vi "Draw Frame.vi"(8 "Error In":errorcluster, 11 "Display In":refnum<class "Display.lvclass">) -> (0 "Error Out":errorcluster, 2 "Frame":u32[][](array[colorbox]), 3 "Display Out":refnum<class "Display.lvclass">)   [LabVIEW 2019, in "Display.lvclass"]
uses:
  Display.lvclass
  Display Element/Display Element.lvclass
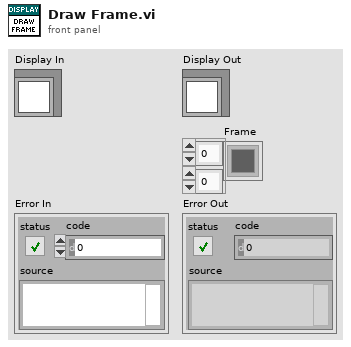
[diagram p1: front panel]
types:
  T1 = typedef "Display Element.lvclass/Pixel.ctl" = cluster{"Position":T2, "Color":u32}
  T2 = typedef "Display Element.lvclass/Vector.ctl" = cluster{"X":i32, "Y":i32}
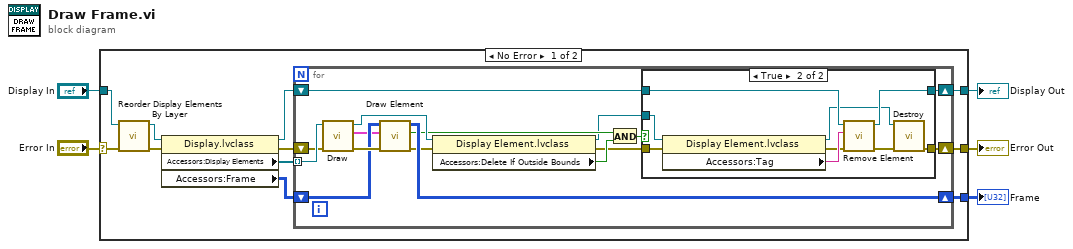
[diagram p0: block diagram]
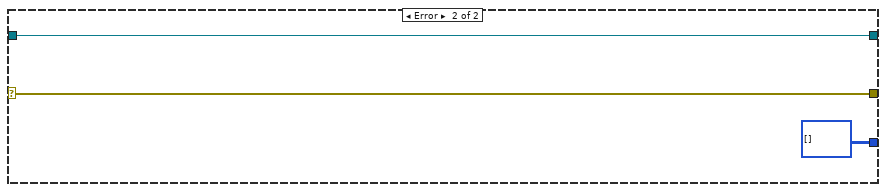
[diagram p3: hidden frame]
diagram:
  n1 = case shown="No Error" "Error In" {
    selector: "Error In" -> [w7 w45]
    tunnel: "Display In" -> [w6 w46]
    tunnel: [w11 w46] -> w3
    tunnel: [w13 w45] -> w2
    tunnel: [w14 u32[][] [] ("Accessors:Frame")] -> w1
    frame No Error {
      n2 = call "Reorder Display Elements By Layer.vi"("Error In"=w7, "Display In"=w6) -> ("Error Out"=w8:errorcluster, "Display Out"=w9:refnum<class "Display.lvclass">)  [unwired: 8 in]
      n3 = property class="Display.lvclass"(reference=w9, error in=w8) -> (reference out=w12:refnum<class "Display.lvclass">, error out=w15:errorcluster, "Accessors:Display Elements"=w16:refnum<class "Display Element.lvclass">[], "Accessors:Frame"=w10:u32[][])
      n4 = for {
        tunnel: w16 -> [w32] mode=indexing
        shift-right: [w28] -> w13
        shift-left: w15 -> [w31]
        shift-right: [w29] -> w14
        shift-left: w10 -> [w25]
        shift-right: [w26] -> w11
        shift-left: w12 -> [w27]
        n5 = call-dynamic "Draw.vi"("Error In"=w31, "Display Element In"=w32) -> ("Error Out"=w30:errorcluster, "Element To Display"=w24:T1[], "Display Element Out"=w23:refnum<class "Display Element.lvclass">)  [unwired: 7 in]
        n6 = call "Draw Element.vi"("Error In"=w30, "Element To Display"=w24, "Frame In"=w25) -> ("Error Out"=w22:errorcluster, "Frame Changed?"=w21:bool, "Frame Out"=w29:u32[][])  [unwired: 6 in]
        n7 = property class="Display Element.lvclass"(reference=w23, error in=w22) -> (reference out=w19:refnum<class "Display Element.lvclass">, error out=w17:errorcluster, "Accessors:Delete If Outside Bounds"=w20:bool)
        n8 = And(x=w21, y=w20) -> (x .and. y?=w18:bool)
        n9 = case shown="True" w18 {
          tunnel: [w33 w42] -> w28
          tunnel: w27 -> [w34 w41]
          tunnel: [w34 w40] -> w26
          tunnel: w19 -> [_ w39]
          tunnel: w17 -> [w33 w38]
          frame False {
          }
          frame True {
            n10 = property class="Display Element.lvclass"(reference=w39, error in=w38) -> (reference out=w37:refnum<class "Display Element.lvclass">, error out=w35:errorcluster, "Accessors:Tag"=w36:string)
            n11 = call "Remove Element.vi"("Error In"=w35, "Element Tag"=w36, "Display In"=w41) -> ("Error Out"=w43:errorcluster, "Display Out"=w40:refnum<class "Display.lvclass">)  [unwired: 7 in]
            n12 = call-dynamic "Destroy.vi"("Error In"=w43, "Display Element In"=w37) -> ("Error Out"=w42:errorcluster)  [unwired: 9 in]
          }
        }
      }
    }
    frame Error {
    }
  }
  "Display Out" <- w3
  "Error Out" <- w2
  "Frame" <- w1
